vi "init.vi"() -> (0 "error out":errorcluster, 3 "notifier out":refnum<notifier>)   [LabVIEW 2015]
uses:
  Type Definitions/vars.ctl
panel:
  in  "vars":T1[](array[typedef])=[{"wait count t"=5000, "wait min"=1000, "wait max"=8000, "stim count t"=0, "stim count n"=0, "d stim"=1000, "d timeout"=5000, "timeout win"=4000, "base temp"=20.0, "stim amps"=[10, -10, 5, -5], "n hit"=0, "n catch"=0, "active"=FALSE, "catch"=FALSE, "stimulus"=FALSE, "reward given"=FALSE, "pairing"=FALSE, "lick"=FALSE, "next reward"=FALSE, "clean tubes"=FALSE, "next temp"=0.0}, {"wait count t"=5000, "wait min"=1000, "wait max"=8000, "stim count t"=0, "stim count n"=0, "d stim"=1000, "d timeout"=5000, "timeout win"=4000, "base temp"=20.0, "stim amps"=[10, -10, 5, -5], "n hit"=0, "n catch"=0, "active"=FALSE, "catch"=FALSE, "stimulus"=FALSE, "reward given"=FALSE, "pairing"=FALSE, "lick"=FALSE, "next reward"=FALSE, "clean tubes"=FALSE, "next temp"=0.0}, {"wait count t"=800, "wait min"=100, "wait max"=800, "stim count t"=0, "stim count n"=0, "d stim"=1000, "d timeout"=5000, "timeout win"=4000, "base temp"=0.0, "stim amps"=[10], "n hit"=0, "n catch"=0, "active"=FALSE, "catch"=FALSE, "stimulus"=FALSE, "reward given"=FALSE, "pairing"=FALSE, "lick"=FALSE, "next reward"=FALSE, "clean tubes"=FALSE, "next temp"=0.0}, {"wait count t"=5000, "wait min"=1000, "wait max"=8000, "stim count t"=0, "stim count n"=0, "d stim"=1000, "d timeout"=5000, "timeout win"=4000, "base temp"=20.0, "stim amps"=[10, -10, 5, -5], "n hit"=0, "n catch"=0, "active"=FALSE, "catch"=FALSE, "stimulus"=FALSE, "reward given"=FALSE, "pairing"=FALSE, "lick"=FALSE, "next reward"=FALSE, "clean tubes"=FALSE, "next temp"=0.0}]
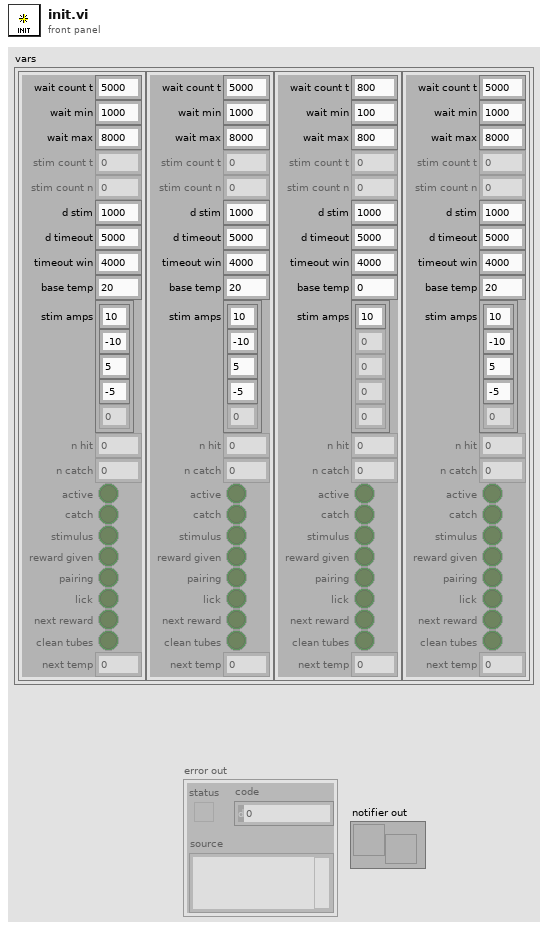
[diagram p1: front panel]
types:
  T1 = typedef "vars.ctl" = cluster{"wait count t":u16, "wait min":u16, "wait max":u16, "stim count t":u16, "stim count n":u16, "d stim":u16, "d timeout":u16, "timeout win":u16, "base temp":sgl, "stim amps":i32[], "n hit":u16, "n catch":u16, "active":bool, "catch":bool, "stimulus":bool, "reward given":bool, "pairing":bool, "lick":bool, "next reward":bool, "clean tubes":bool, "next temp":sgl}
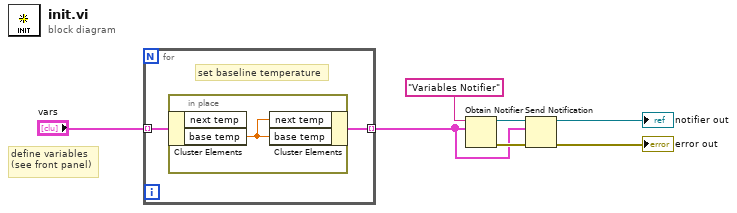
[diagram p0: block diagram]
diagram:
  # "define variables\n(see front panel)"
  n1 = for {
    tunnel: "vars" -> [w9] mode=indexing
    tunnel: [w8] -> w2 mode=indexing
    # "set baseline temperature"
    n2 = in-place {
      n3 = in-place-cluster #1(w9) -> ("base temp"=w10:sgl)  [unwired: 1 out]
      n4 = in-place-cluster #1("next temp"=w10, "base temp"=w10) -> (w8:T1)
    }
  }
  n5 = Obtain Notifier(name (unnamed)="Variables Notifier", notification data type=w2) -> (notifier out=w6:refnum<notifier>, error out=w5:errorcluster)  [unwired: 2 in, 1 out]
  n6 = Send Notification(notification=w2, notifier=w6, error in (no error)=w5) -> (notifier out=→"notifier out":refnum<notifier>, error out=→"error out":errorcluster)
